vi "Configure Signaling RF UL Channel Number A.vi"(8 "error in (no error)":errorcluster, 9 "UL Channel Number A (0)":i32, 10 "Cell Name (\"Cell Name\")":string="Cell Name", 11 "VISA resource name":refnum<visa-resource-name>) -> (0 "error out":errorcluster, 3 "VISA resource name out":refnum<visa-resource-name>)   [LabVIEW 2020, in "Rohde&Schwarz CMWXP NR FR1 Measurement.lvlib"]
doc: "Sets the user-defined channel number of point A, for the uplink.\n\nAttribute:\nRSCMWXPNRFR1M_ATTR_SIGNALING_RF_UL_CHANNEL_NUMBER_A\n\nRemote-control command:\n[CONFigure:]SIGNaling:NRADio:CELL:RFSettings:UL:APOint:ARFCn"
uses:
  <instrlib>/Rohde&Schwarz CMWXP NR FR1 Measurement/Rohde&Schwarz CMWXP NR FR1 Measurement.lvlib
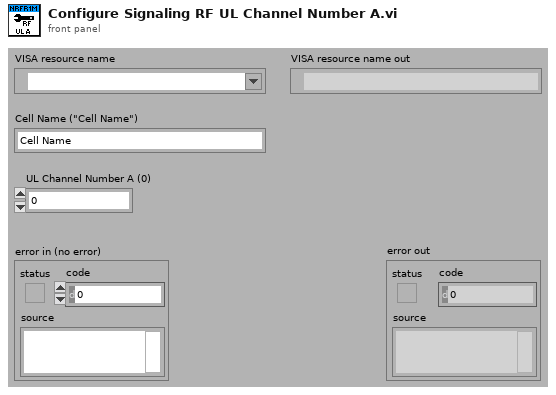
[diagram p1: front panel]
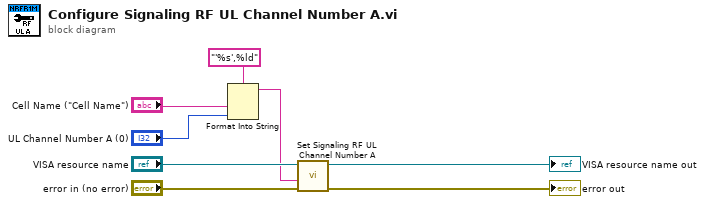
[diagram p0: block diagram]
diagram:
  n1 = Format Into String(format string="'%s',%ld", "Cell Name (\"Cell Name\")", "UL Channel Number A (0)") -> (resulting string=w1:string)  [unwired: 2 in, 1 out]
  n2 = call "Set Signaling RF UL Channel Number A"("error in (no error)"="error in (no error)", "Signaling RF UL Channel Number A ()"=w1, "instrument handle"="VISA resource name") -> ("error out"=→"error out":errorcluster, "instrument handle out"=→"VISA resource name out":refnum<visa-resource-name>)  [unwired: 7 in]
